vi "Log Replace Array Subset.vi"(8 "new subarray":dbl[](array[numeric]), 9 "values index":i32, 10 "values array":dbl[](array[numeric]), 11 "log file":path=path "c:/ni-rt/VeriStand/Custom Devices/Rx Read From Hardware Replace Parameters.txt") -> ()   [LabVIEW 2020]
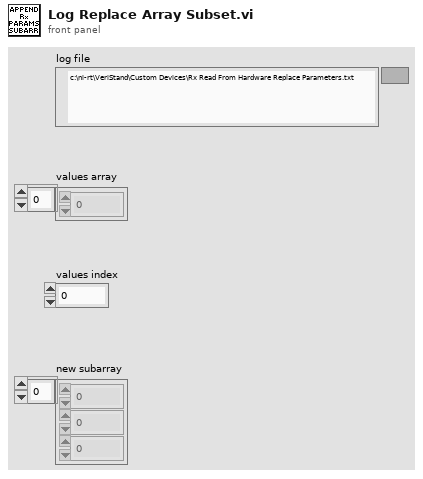
[diagram p1: front panel]
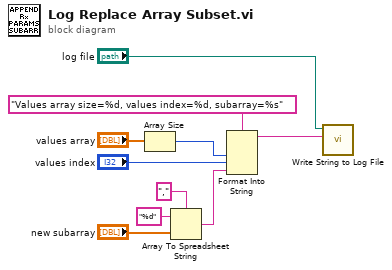
[diagram p0: block diagram]
diagram:
  n1 = Array Size(array="values array") -> (size(s)=w9:i32)
  n2 = Array To Spreadsheet String(delimiter (Tab)=",", array="new subarray", 3:"%d" ("format string")) -> (spreadsheet string=w4:string)
  n3 = Format Into String(format string="Values array size=%d, values index=%d, subarray=%s", w9, "values index", w4) -> (resulting string=w2:string)  [unwired: 2 in, 1 out]
  n4 = call "Write String to Log File.vi"("string to log"=w2, "log file"="log file") -> ()  [unwired: 9 in, 1 out]
